vi "lectura.vi"() -> ()   [LabVIEW 2020]
panel:
  out "Waveform Graph":dbl[](graph)
  in  "DETENER":bool
  out "ALARMA":bool
  out "LIMITE":dbl
  out "Waveform Chart":dynamicdata(graph)
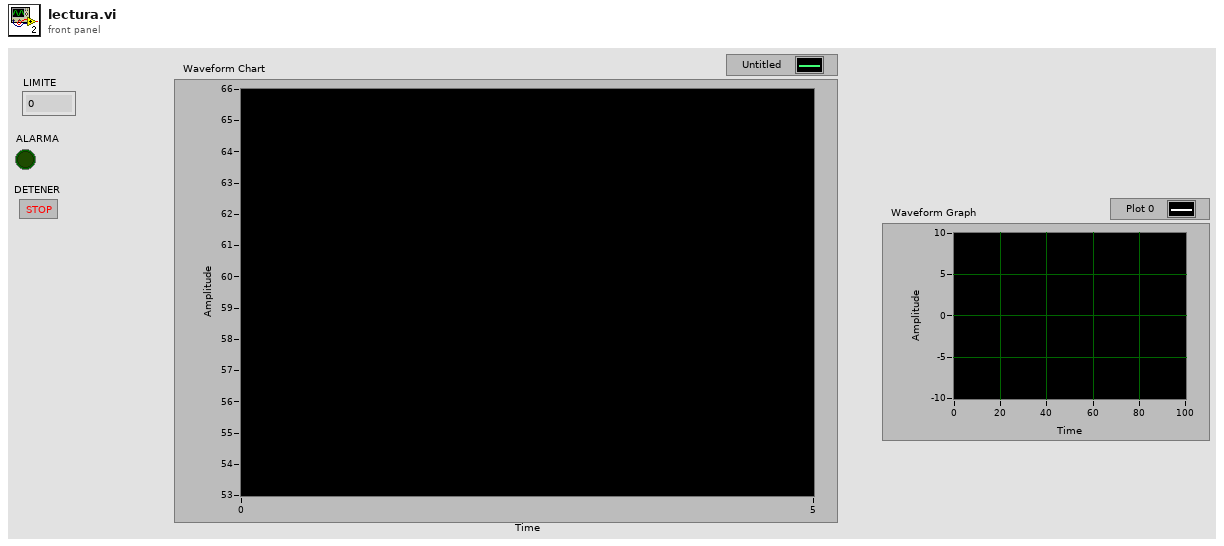
[diagram p1: front panel]
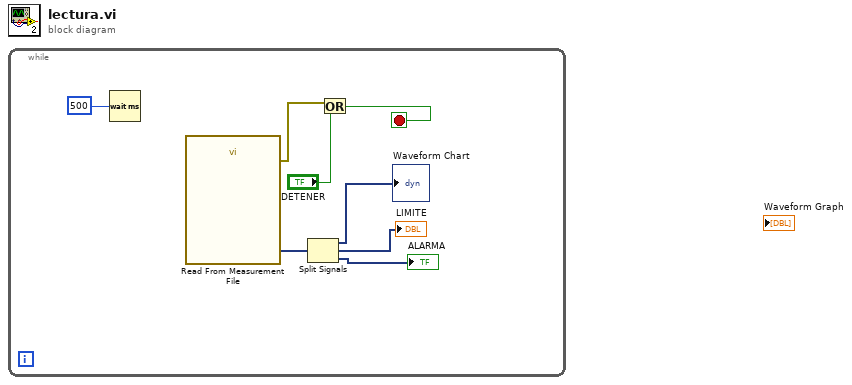
[diagram p0: block diagram]
diagram:
  n1 = while {
    stop <- w5 stop-if-true
    n2 = Wait (ms)(milliseconds to wait=u32 500 ("millisecond timer value")) -> ()  [unwired: 1 out]
    n3 = call "Read From Measurement File"() -> ("error out"=w7:errorcluster, "Signals"=w2:dynamicdata)  [unwired: 6 in, 4 out]
    n4 = Split Signals(w2) -> (→"Waveform Chart":dynamicdata, →"LIMITE":dynamicdata, →"ALARMA":dynamicdata)  [unwired: 3 in]
    n5 = Or(x=w7, y="DETENER") -> (x .or. y?=w5:bool)
  }
